vi "addDocumentElement.vi"(7 "Name":string, 8 "error in (no error)":errorcluster, 9 "Value":refnum<class "tBSONDocument.lvclass">, 10 "Replace? (false)":bool, 11 "tBSONDocument in":refnum<class "tBSONDocument.lvclass">) -> (0 "error out":errorcluster, 3 "tBSONDocument out":refnum<class "tBSONDocument.lvclass">)   [LabVIEW 2013, in "BSON.lvlib" / "tBSONDocument.lvclass"]
doc: "Adds a BSON document as an element to a BSON document."
uses:
  tBSONDocument.lvclass
  BSONElements/tBSONDocumentElement/tBSONDocumentElement.lvclass
  tBSONElement/tBSONElement.lvclass
  tBSONElement/setName.vi
  BSONElements/tBSONDocumentElement/setValue.vi
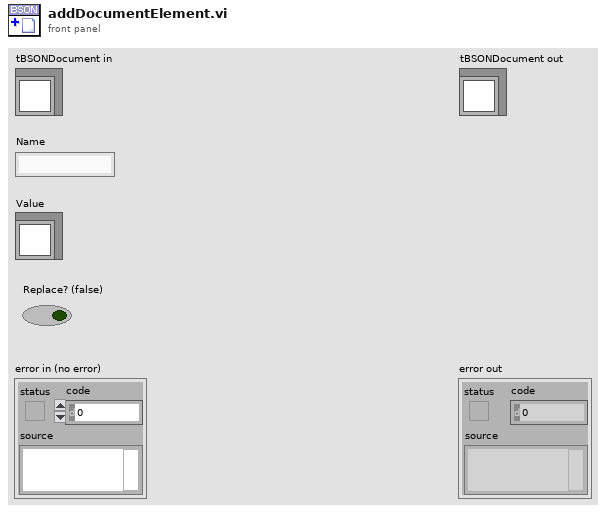
[diagram p1: front panel]
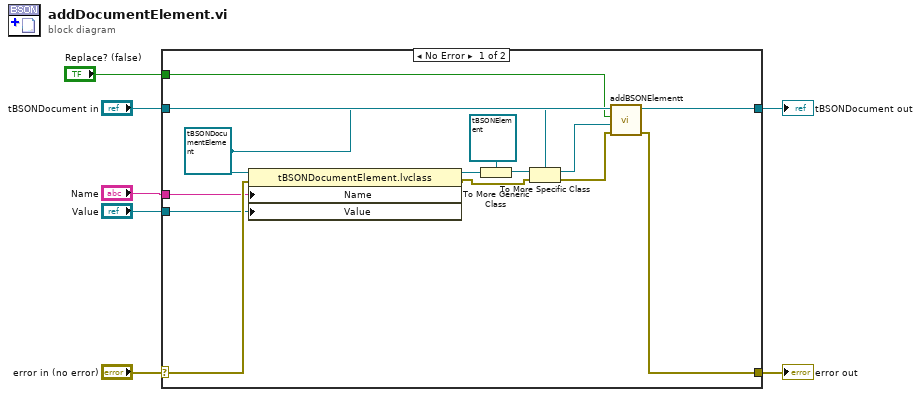
[diagram p0: block diagram]
diagram:
  n1 = case shown="No Error" "error in (no error)" {
    selector: "error in (no error)" -> [w21 w23]
    tunnel: [w15 w23] -> w6
    tunnel: [w16 w22] -> w4
    tunnel: "tBSONDocument in" -> [w17 w22]
    tunnel: "Name" -> [w14 _]
    tunnel: "Value" -> [w20 _]
    tunnel: "Replace? (false)" -> [w8 _]
    frame No Error {
      w10 = refnum<class "tBSONDocumentElement.lvclass"> refnum ("BSON.lvlib:tBSONDocumentElement.lvclass")
      n2 = property class="tBSONDocumentElement.lvclass"(reference=w10, error in=w21, "Name"=w14, "Value"=w20) -> (reference out=w19:refnum<class "tBSONDocumentElement.lvclass">, error out=w13:errorcluster)
      n3 = To More Generic Class(target class=refnum<class "tBSONElement.lvclass"> refnum ("BSON.lvlib:tBSONElement.lvclass"), reference=w19) -> (generic class reference=w12:refnum<class "tBSONElement.lvclass">)
      n4 = To More Specific Class(target class=w10, reference=w12, error in=w13) -> (specific class reference=w11:refnum<class "tBSONDocumentElement.lvclass">, error out=w9:errorcluster)
      n5 = call "addBSONElementt.vi"("error in (no error)"=w9, "Element"=w11, "Replace? (false)"=w8, "tBSONDocument in"=w17) -> ("error out"=w15:errorcluster, "tBSONDocument out"=w16:refnum<class "tBSONDocument.lvclass">)  [unwired: 6 in]
    }
    frame Error {
    }
  }
  "error out" <- w6
  "tBSONDocument out" <- w4
